vi "gen_PES_MELEXIR.vi"(0 "Img Data":T2, 2 "Current VI's Path":path, 7 "PES Data In":cluster{"Pixel":dbl[], "Intensity":dbl[]}, 11 "Controls":T1, 12 "Elapsed Time / ms":u32) -> (4 "Img Data Out":T2, 8 "PES Data":cluster{"Pixel":dbl[], "Intensity":dbl[]}, 14 "Elapsed Time / ms Out":u32, 15 "Controls Out":T1)   [LabVIEW 2023]
panel:
  out "error out":errorcluster
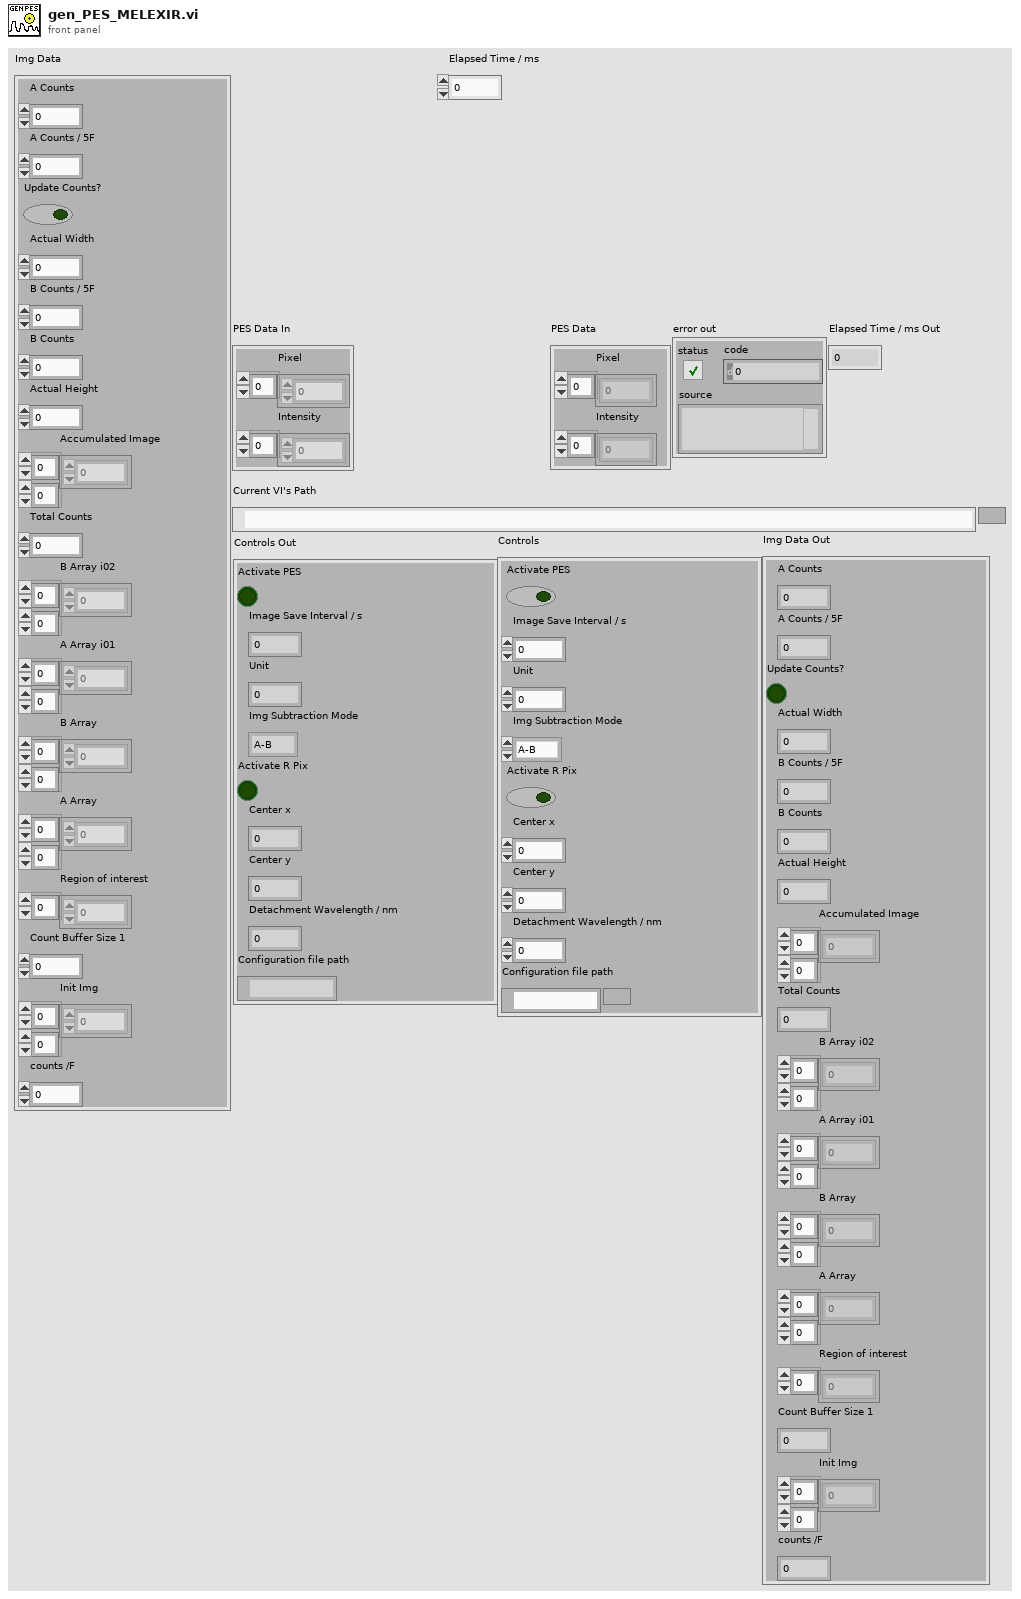
[diagram p1: front panel]
types:
  T1 = cluster{"Activate PES":bool, "Image Save Interval / s":dbl, "Unit":u16, "Img Subtraction Mode":enum16{"A-B", "B-A", "A+B"}, "Activate R Pix":bool, "Center x":i32, "Center y":i32, "Detachment Wavelength / nm":dbl, "Configuration file path":path}
  T2 = cluster{"A Counts":i32, "A Counts / 5F":dbl, "Update Counts?":bool, "Actual Width":u32, "B Counts / 5F ":dbl, "B Counts":i32, "Actual Height":u32, "Accumulated Image ":i16[][], "Total Counts":i32, "B Array i02":sgl[][], "A Array i01":sgl[][], "B Array":i16[][], "A Array":i16[][], "Region of interest":i32[], "Count Buffer Size 1":i32, "Init Img":i16[][], "counts /F":i16}
  T3 = cluster{"Electron Kinetic Energy / eV":dbl[], "Binding Energy / eV":dbl[], "Pixel":dbl[], "Intensity":dbl[]}
  T4 = cluster{"Electron Kinetic Energy / eV":dbl[], "Intensity":dbl[]}
  T5 = cluster{"Binding Energy / eV":dbl[], "Intensity":dbl[]}
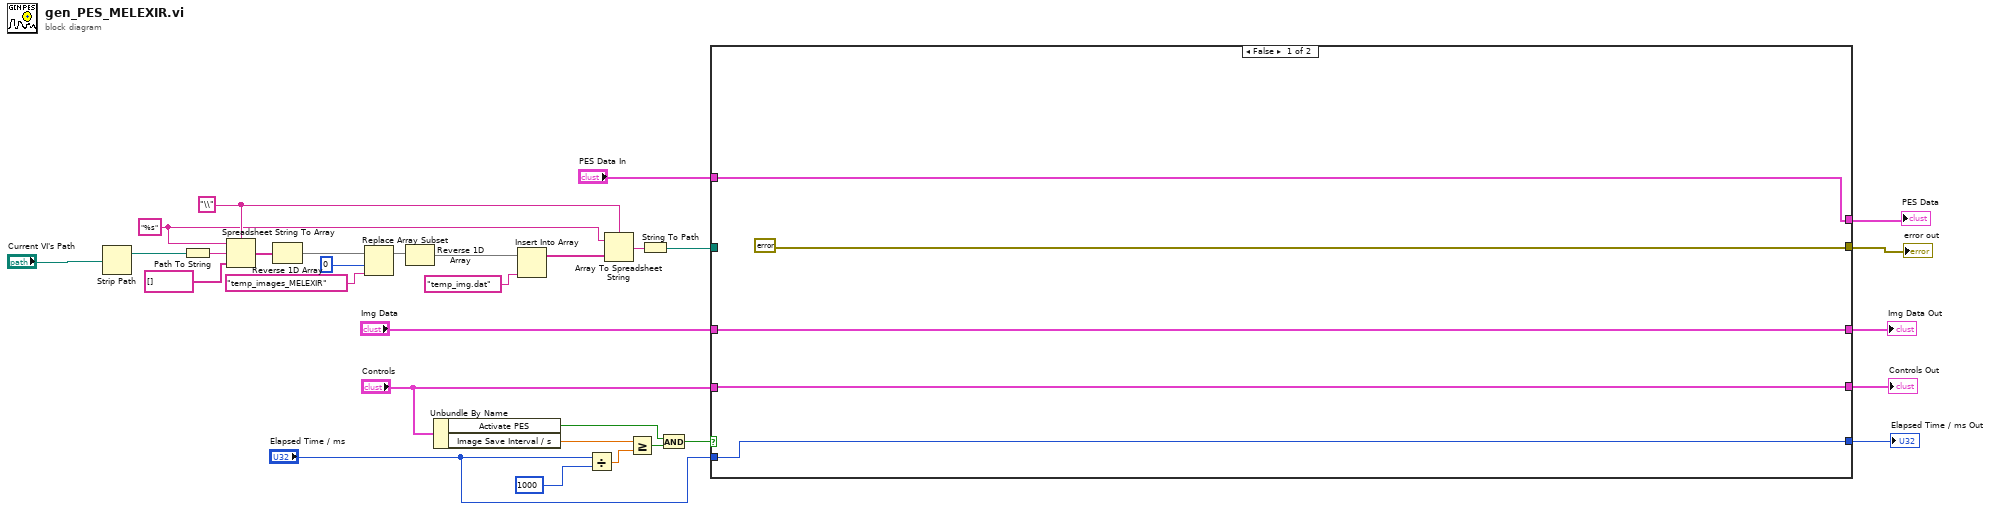
[diagram p0: block diagram]
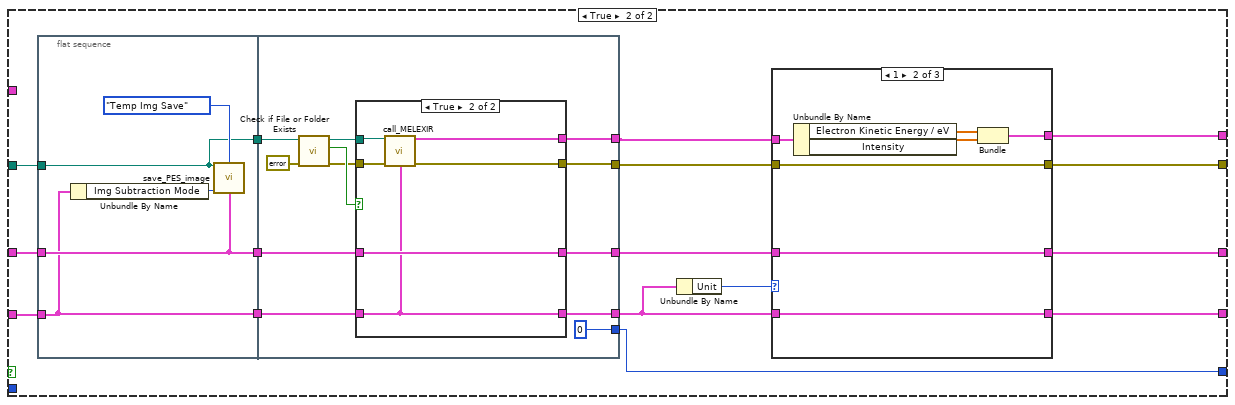
[diagram p2: hidden frame]
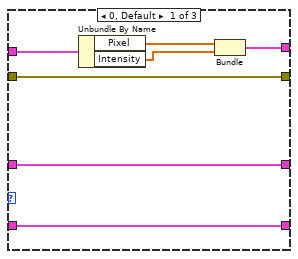
[diagram p3: hidden frame]
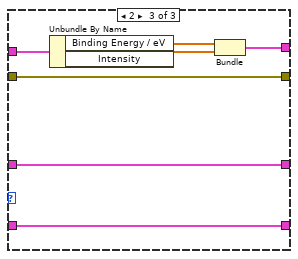
[diagram p4: hidden frame]
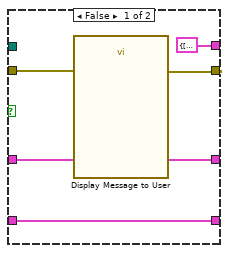
[diagram p5: hidden frame]
diagram:
  w12 = "%s" ("format string")
  w13 = "\\" ("delimiter (Tab)")
  n1 = Strip Path(path="Current VI's Path") -> (stripped path=w18:path)  [unwired: 1 out]
  n2 = Path To String(path=w18) -> (string=w19:string)
  n3 = Spreadsheet String To Array(delimiter (Tab)=w13, format string=w12, spreadsheet string=w19, array type (2D Dbl)=string[] [] ("appended array")) -> (array=w20:string[])
  n4 = Reverse 1D Array(array=w20) -> (reversed array=w21:string[])
  n5 = Replace Array Subset(array=w21, new element="temp_images_MELEXIR" ("new element/subarray"), index=0) -> (w22:string[])
  n6 = Reverse 1D Array(array=w22) -> (reversed array=w23:string[])
  n7 = Unbundle By Name("Controls") -> ("Activate PES"=w27:bool, "Image Save Interval / s"=w31:dbl)
  n8 = Insert Into Array(array=w23, new element="temp_img.dat" ("new element/subarray")) -> (w24:string[])  [unwired: 1 in]
  n9 = Divide(x="Elapsed Time / ms", y=u32 1000) -> (x/y=w29:dbl)
  n10 = Array To Spreadsheet String(delimiter (Tab)=w13, array=w24, 3:w12) -> (spreadsheet string=w10:string)
  n11 = Greater Or Equal?(x=w31, y=w29) -> (x >= y?=w28:bool)
  n12 = String To Path(string=w10) -> (path=w9:path)
  n13 = And(x=w27, y=w28) -> (x .and. y?=w26:bool)
  n14 = case shown="False" w26 {
    tunnel: "Img Data" -> [w32 w52]
    tunnel: "Controls" -> [w34 w51]
    tunnel: "Elapsed Time / ms" -> [w33 _]
    tunnel: w9 -> [_ w48]
    tunnel: "PES Data In" -> [w35 _]
    tunnel: [w35 w42] -> w5
    tunnel: [errorcluster {"status"=FALSE, "code"=0, "source"=""} ("error out") w41] -> w4
    tunnel: [w34 w40] -> w3
    tunnel: [w33 w39] -> w2
    tunnel: [w32 w37] -> w1
    frame False {
    }
    frame True {
      n15 = flat-sequence {
        tunnel: w52 -> [w78]
        tunnel: w51 -> [w76]
        tunnel: [w78] -> w50
        tunnel: [w76] -> w49
        tunnel: w48 -> [w74]
        tunnel: [w74] -> w47
        tunnel: w50 -> [w90]
        tunnel: w49 -> [w89]
        tunnel: w47 -> [w84]
        tunnel: [w88] -> w38
        tunnel: [w87] -> w43
        tunnel: [w83] -> w45
        tunnel: [u32 0 ("Elapsed Time / ms")] -> w39
        tunnel: [w81] -> w44
        frame #0 {
          n16 = Unbundle By Name(w76) -> ("Img Subtraction Mode"=w75:enum16{"A-B", "B-A", "A+B"})
          n17 = call "save_PES_image.vi"("Temp Save Path"=w74, "Save Type"=enum16{"Temp Img Save", "Custom Save"}."Temp Img Save", "Img Subtraction Mode"=w75, "Image Data In"=w78) -> ()  [unwired: 12 in]
        }
        frame #1 {
          n18 = call <vilib>:"Check if File or Folder Exists.vi"("error in (no error)"=errorcluster {"status"=FALSE, "code"=0, "source"=""}, "path"=w84) -> ("error out"=w85:errorcluster, "file or folder exists?"=w86:bool, "dup path"=w80:path)  [unwired: 7 in]
          n19 = case shown="True" w86 {
            tunnel: w90 -> [w95 w101]
            tunnel: w89 -> [w94 w97]
            tunnel: [w95 w101] -> w88
            tunnel: [w94 w97] -> w87
            tunnel: w85 -> [w93 w100]
            tunnel: w80 -> [_ w96]
            tunnel: [w92 w99] -> w81
            tunnel: [T3 {"Electron Kinetic Energy / eV"=[], "Binding Energy / eV"=[], "Pixel"=[], "Intensity"=[]} ("PES Data Out") w98] -> w83
            frame False {
              n20 = call "Display Message to User"("error in (no error)"=w93) -> ("error out"=w92:errorcluster)  [unwired: 9 in, 1 out]
            }
            frame True {
              n21 = call "call_MELEXIR.vi"("Image Proc Directory"=w96, "error in (no error)"=w100, "Controls"=w97) -> ("PES Data Out"=w98:T3, "error out"=w99:errorcluster)  [unwired: 11 in]
            }
          }
        }
      }
      n22 = Unbundle By Name(w43) -> ("Unit"=w46:u16)
      n23 = case shown="1" w46 {
        tunnel: w45 -> [w59 w66 w73]
        tunnel: [w56 w63 w70] -> w42
        tunnel: w44 -> [w55 w62 w69]
        tunnel: [w55 w62 w69] -> w41
        tunnel: w43 -> [w54 w61 w68]
        tunnel: [w54 w61 w68] -> w40
        tunnel: w38 -> [w53 w60 w67]
        tunnel: [w53 w60 w67] -> w37
        frame 0, Default {
          n24 = Unbundle By Name(w59) -> ("Pixel"=w58:dbl[], "Intensity"=w57:dbl[])
          n25 = Bundle("Pixel"=w58, "Intensity"=w57) -> (w56:cluster{"Pixel":dbl[], "Intensity":dbl[]})  [unwired: 1 in]
        }
        frame 1 {
          n26 = Unbundle By Name(w66) -> ("Electron Kinetic Energy / eV"=w65:dbl[], "Intensity"=w64:dbl[])
          n27 = Bundle("Electron Kinetic Energy / eV"=w65, "Intensity"=w64) -> (w63:T4)  [unwired: 1 in]
        }
        frame 2 {
          n28 = Unbundle By Name(w73) -> ("Binding Energy / eV"=w72:dbl[], "Intensity"=w71:dbl[])
          n29 = Bundle("Binding Energy / eV"=w72, "Intensity"=w71) -> (w70:T5)  [unwired: 1 in]
        }
      }
    }
  }
  "PES Data" <- w5
  "error out" <- w4
  "Controls Out" <- w3
  "Elapsed Time / ms Out" <- w2
  "Img Data Out" <- w1
